vi "save.vi"(8 "error in (no error)":errorcluster, 11 "TrajectoryDL091126GenericVoxel in":refnum<class "TrajectoryDL091126GenericVoxel.lvclass">) -> (0 "error out":errorcluster, 3 "TrajectoryDL091126GenericVoxel out":refnum<class "TrajectoryDL091126GenericVoxel.lvclass">)   [LabVIEW 2010, in "TrajectoryDL091126GenericVoxel.lvclass"]
doc: "saves the trajectory coordinates and the corresponding intensity values into separate files"
uses:
  TrajectoryDL091126GenericVoxel.lvclass
  common/enumerations/x_y_z_enumeration.ctl
  common/enumerations/functional_global_action_enum.ctl
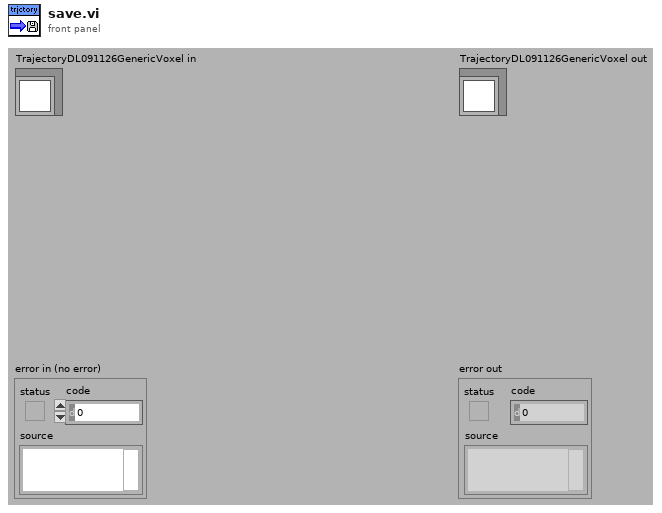
[diagram p1: front panel]
types:
  T1 = typedef "x_y_z_enumeration.ctl" = enum16{"x", "y", "z"}
  T2 = typedef "functional_global_action_enum.ctl" = enum16{"get", "set", "reset"}
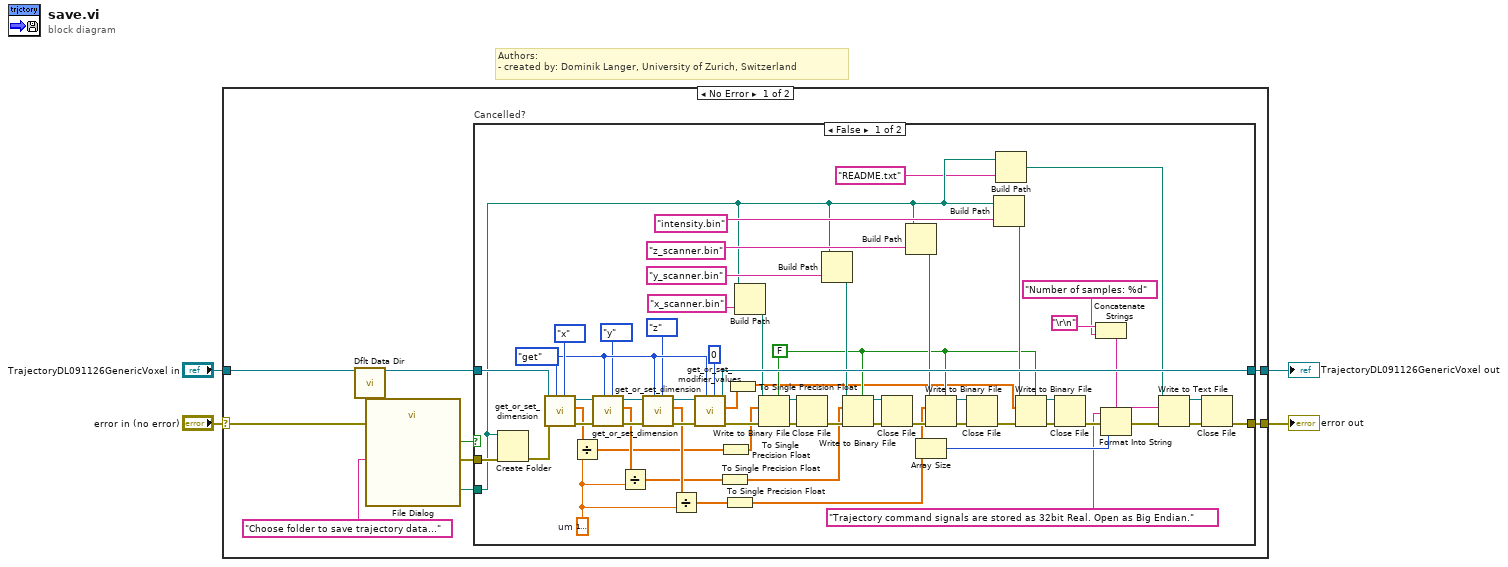
[diagram p0: block diagram]
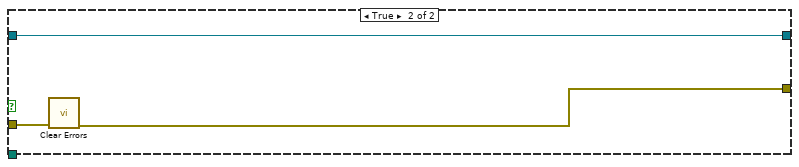
[diagram p2: hidden frame]
diagram:
  # "Authors: \n- created by: Dominik Langer, University of Zurich, Switzerland"
  n1 = case shown="No Error" "error in (no error)" {
    selector: "error in (no error)" -> [w11 w80]
    tunnel: [w8 w80] -> w3
    tunnel: [w12 w79] -> w1
    tunnel: "TrajectoryDL091126GenericVoxel in" -> [w13 w79]
    frame No Error {
      n2 = call <vilib>:"Dflt Data Dir.vi"() -> ("App:Default Data Directory"=w6:path)
      n3 = call "File Dialog"("start path"=w6, "prompt"="Choose folder to save trajectory data...", "error in"=w11) -> ("selected path"=w9:path, "cancelled"=w7:bool, "error out"=w10:errorcluster)  [unwired: 9 in, 1 out]
      n4 = case "Cancelled?" shown="False" w7 {
        tunnel: w13 -> [w69 w76]
        tunnel: [w68 w76] -> w12
        tunnel: w10 -> [w37 w78]
        tunnel: w9 -> [w35 _]
        tunnel: [w30 w77] -> w8
        frame False {
          w38 = FALSE ("prepend array or string size? (T)")
          w59 = dbl[unit] 1e-06  # um
          w66 = functional_global_action_enum."get" ("action")
          n5 = Create Folder(path (use dialog)=w35, error in=w37) -> (error out=w36:errorcluster)  [unwired: 1 in, 2 out]
          n6 = call-dynamic "get_or_set_dimension.vi"("dimension"=x_y_z_enumeration."x", "action"=w66, "error in (no error)"=w36, "GenericTrajectory in"=w69) -> ("error out"=w71:errorcluster, "pixel values out (single dimension)"=w62:dbl[unit][], "GenericTrajectory out"=w74:refnum<class "TrajectoryDL091126GenericVoxel.lvclass">)  [unwired: 5 in]
          n7 = Divide(x=w62, y=w59) -> (x/y=w21:dbl[])
          n8 = call-dynamic "get_or_set_dimension.vi"("dimension"=x_y_z_enumeration."y", "action"=w66, "error in (no error)"=w71, "GenericTrajectory in"=w74) -> ("error out"=w75:errorcluster, "pixel values out (single dimension)"=w61:dbl[unit][], "GenericTrajectory out"=w73:refnum<class "TrajectoryDL091126GenericVoxel.lvclass">)  [unwired: 5 in]
          n9 = Divide(x=w61, y=w59) -> (x/y=w19:dbl[])
          n10 = call-dynamic "get_or_set_dimension.vi"("dimension"=x_y_z_enumeration."z", "action"=w66, "error in (no error)"=w75, "GenericTrajectory in"=w73) -> ("error out"=w72:errorcluster, "pixel values out (single dimension)"=w60:dbl[unit][], "GenericTrajectory out"=w70:refnum<class "TrajectoryDL091126GenericVoxel.lvclass">)  [unwired: 5 in]
          n11 = Divide(x=w60, y=w59) -> (x/y=w17:dbl[])
          n12 = call-dynamic "get_or_set_modifier_values.vi"("modifier index"=0, "action"=w66, "error in (no error)"=w72, "GenericTrajectory in"=w70) -> ("error out"=w50:errorcluster, "modifier values out"=w15:dbl[], "GenericTrajectory out"=w68:refnum<class "TrajectoryDL091126GenericVoxel.lvclass">)  [unwired: 5 in]
          n13 = To Single Precision Float(number=w19) -> (single precision float=w18:sgl[])
          n14 = To Single Precision Float(number=w21) -> (single precision float=w20:sgl[])
          n15 = To Single Precision Float(number=w17) -> (single precision float=w16:sgl[])
          n16 = To Single Precision Float(number=w15) -> (single precision float=w14:sgl[])
          n17 = Build Path(base path=w35, name or relative path="x_scanner.bin") -> (appended path=w57:path)
          n18 = Write to Binary File(file (use dialog)=w57, data=w20, error in=w50, 5:w38) -> (refnum out=w49:refnum<file>, error out=w48:errorcluster)  [unwired: 2 in, 1 out]
          n19 = Close File(refnum=w49, error in=w48) -> (error out=w47:errorcluster)  [unwired: 1 out]
          n20 = Build Path(base path=w35, name or relative path="y_scanner.bin") -> (appended path=w56:path)
          n21 = Write to Binary File(file (use dialog)=w56, data=w18, error in=w47, 5:w38) -> (refnum out=w40:refnum<file>, error out=w41:errorcluster)  [unwired: 2 in, 1 out]
          n22 = Close File(refnum=w40, error in=w41) -> (error out=w39:errorcluster)  [unwired: 1 out]
          n23 = Build Path(base path=w35, name or relative path="z_scanner.bin") -> (appended path=w54:path)
          n24 = Array Size(array=w16) -> (size(s)=w26:i32)
          n25 = Write to Binary File(file (use dialog)=w54, data=w16, error in=w39, 5:w38) -> (refnum out=w44:refnum<file>, error out=w43:errorcluster)  [unwired: 2 in, 1 out]
          n26 = Close File(refnum=w44, error in=w43) -> (error out=w42:errorcluster)  [unwired: 1 out]
          n27 = Build Path(base path=w35, name or relative path="intensity.bin") -> (appended path=w53:path)
          n28 = Build Path(base path=w35, name or relative path="README.txt") -> (appended path=w33:path)
          n29 = Write to Binary File(file (use dialog)=w53, data=w14, error in=w42, 5:w38) -> (refnum out=w46:refnum<file>, error out=w45:errorcluster)  [unwired: 2 in, 1 out]
          n30 = Close File(refnum=w46, error in=w45) -> (error out=w29:errorcluster)  [unwired: 1 out]
          n31 = Concatenate Strings("\r\n", "Number of samples: %d" ("string")) -> (w23:string)
          n32 = Format Into String(format string=w23, initial string="Trajectory command signals are stored as 32bit Real. Open as Big Endian." ("text"), error in=w29, w26) -> (resulting string=w27:string, error out=w28:errorcluster)
          n33 = Write to Text File(file (use dialog)=w33, text=w27, error in=w28) -> (refnum out=w32:refnum<file>, error out=w31:errorcluster)  [unwired: 1 in, 1 out]
          n34 = Close File(refnum=w32, error in=w31) -> (error out=w30:errorcluster)  [unwired: 1 out]
        }
        frame True {
          n35 = call <vilib>:"Clear Errors.vi"("error in (no error)"=w78) -> ("error out"=w77:errorcluster)  [unwired: 6 in]
        }
      }
    }
    frame Error {
    }
  }
  "error out" <- w3
  "TrajectoryDL091126GenericVoxel out" <- w1
